vi "RayTriangleIntersection.vi"(10 "Ray":T1, 11 "TriangleFace":T2) -> (1 "Intersects":bool, 2 "P0":cluster{"X":dbl, "Y":dbl, "Z":dbl}, 3 "r":dbl)   [LabVIEW 2014]
uses:
  TypeDefs/TriangleFace.ctl
  TypeDefs/Point3D.ctl
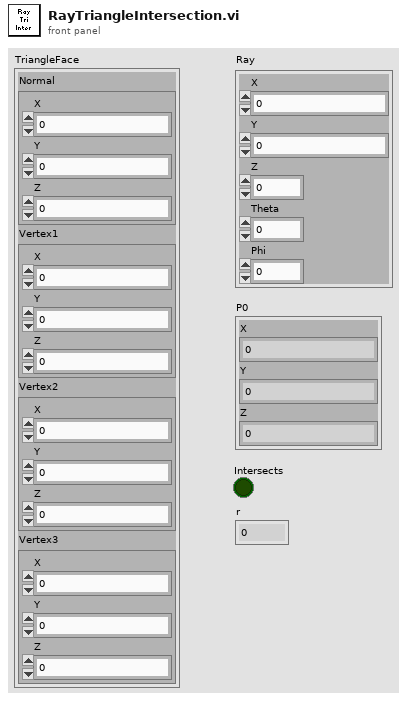
[diagram p1: front panel]
types:
  T1 = cluster{"X":dbl, "Y":dbl, "Z":dbl, "Theta":dbl, "Phi":dbl}
  T2 = typedef "TriangleFace.ctl" = cluster{"Normal":T3, "Vertex1":T3, "Vertex2":T3, "Vertex3":T3}
  T3 = typedef "Point3D.ctl" = cluster{"X":sgl, "Y":sgl, "Z":sgl}
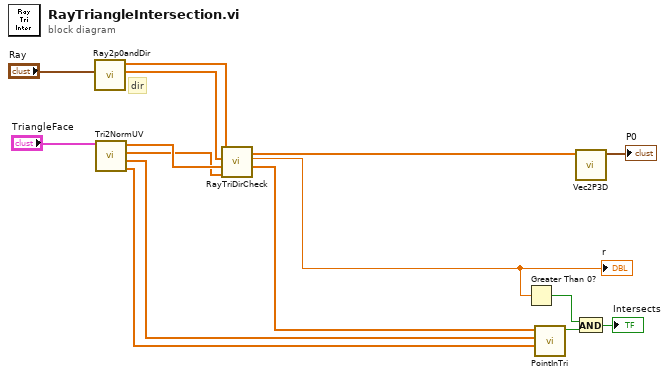
[diagram p0: block diagram]
diagram:
  # "dir"
  n1 = call "Ray2p0andDir.vi"("Ray"="Ray") -> ("Dir"=w7:dbl[], "P0"=w13:dbl[])  [unwired: 9 in]
  n2 = call "Tri2NormUV.vi"("TriangleFace"="TriangleFace") -> ("v"=w1:dbl[], "u"=w11:dbl[], "Normal"=w6:dbl[], "TriVertex"=w12:dbl[])  [unwired: 7 in]
  n3 = call "RayTriDirCheck.vi"("Normal"=w6, "TriVertex"=w12, "Dir"=w7, "P0"=w13) -> ("w"=w10:dbl[], "r"=w3:dbl, "I"=w9:dbl[])  [unwired: 5 in]
  "r" <- w3
  n4 = Greater Than 0?(x=w3) -> (x > 0?=w2:bool)
  n5 = call "PointInTri.vi"("v"=w1, "u"=w11, "w"=w10) -> ("PointInTri"=w5:bool)  [unwired: 8 in]
  n6 = call "Vec2P3D.vi"("Vec"=w9) -> ("P0"=→"P0":cluster{"X":dbl, "Y":dbl, "Z":dbl})  [unwired: 10 in]
  n7 = And(x=w2, y=w5) -> (x .and. y?=→"Intersects":bool)
